vi "Configure Measurement Trigger Parameters.vi"(8 "error in (no error)":errorcluster, 10 "Trigger Measurement Operation (0: Continuity)":i32(ring) items=["Continuity", "Diode", "Voltage DC Ratio", "Current AC", "Current DC", "Temperature", "Frequency", "Period", "Voltage AC", "Voltage DC", "Resistance 2-wire", "Resistance 4-wire"], 11 "VISA resource name":refnum<visa-resource-name>) -> (0 "error out":errorcluster, 3 "VISA resource name out":refnum<visa-resource-name>)   [LabVIEW 2013, in "Agilent 3446X Series.lvlib"]
doc: "Configures measurement and trigger parameters to their defalt value."
uses:
  Agilent 3446X Series.lvlib
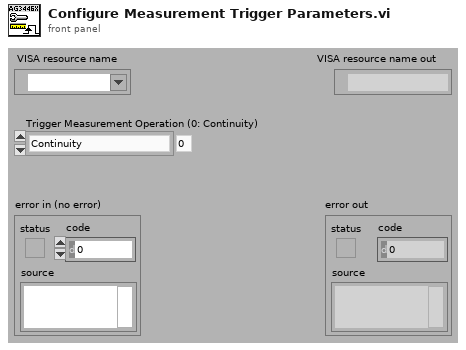
[diagram p1: front panel]
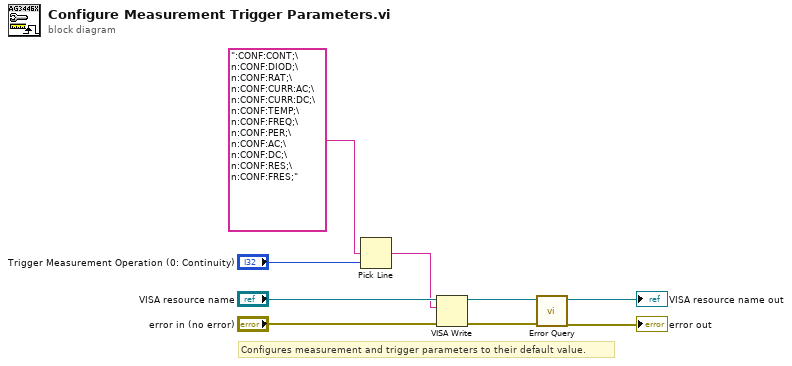
[diagram p0: block diagram]
diagram:
  # "Configures measurement and trigger parameters to their default value."
  n1 = Pick Line(multi-line string=":CONF:CONT;\n:CONF:DIOD;\n:CONF:RAT;\n:CONF:CURR:AC;\n:CONF:CURR:DC;\n:CONF:TEMP;\n:CONF:FREQ;\n:CONF:PER;\n:CONF:AC;\n:CONF:DC;\n:CONF:RES;\n:CONF:FRES;", line index="Trigger Measurement Operation (0: Continuity)") -> (output string=w1:string)  [unwired: 1 in]
  n2 = VISA Write(VISA resource name="VISA resource name", write buffer=w1, error in (no error)="error in (no error)") -> (VISA resource name out=w7:refnum<visa-resource-name>, error out=w6:errorcluster)  [unwired: 1 out]
  n3 = call "Error Query.vi"("error in (no error)"=w6, "VISA resource name"=w7) -> ("error out"=→"error out":errorcluster, "VISA resource name out"=→"VISA resource name out":refnum<visa-resource-name>)  [unwired: 8 out]
